vi "AOTF_NonLinKillTasks.vi"(0 "Refnum in":refnum<k21>, 1 "task out":refnum<k21>, 2 "LineOnOff[3]":bool, 3 "task out 3":refnum<k21>, 4 "LineOnOff[4]":bool, 5 "task out 7":refnum<k21>, 6 "task out 4":refnum<k21>, 7 "error in (no error)":errorcluster, 8 "LineOnOff[2]":bool, 9 "task out 6":refnum<k21>, 10 "task out 2":refnum<k21>, 11 "LineOnOff[0]":bool, 12 "LineOnOff[1]":bool, 13 "LineOnOff[5]":bool, 14 "task out 5":refnum<k21>, 15 "405Pico":refnum<k21>, 16 "LineOnOff[6]":bool, 18 "LineOnOff[7]":bool) -> (27 "error out":errorcluster)   [LabVIEW 2011]
uses:
  Variables/405Pico.vi
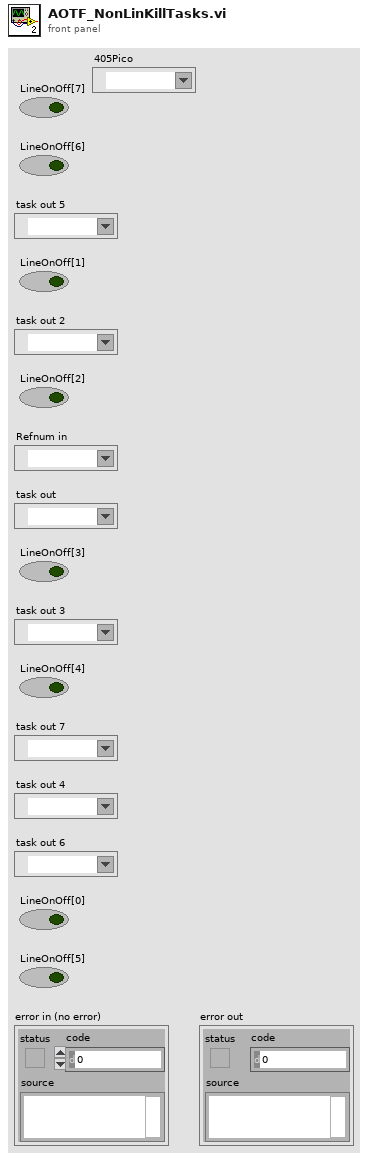
[diagram p1: front panel]
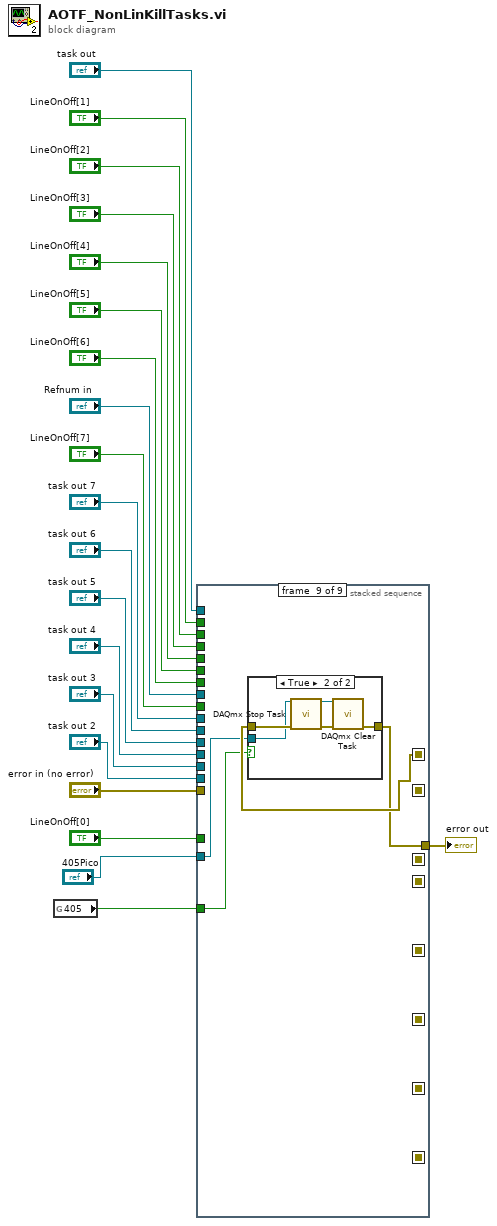
[diagram p0: block diagram]
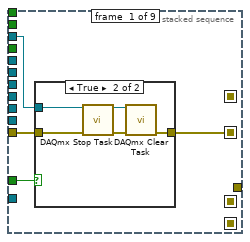
[diagram p2: hidden frame]
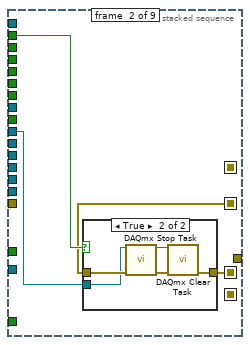
[diagram p4: hidden frame]
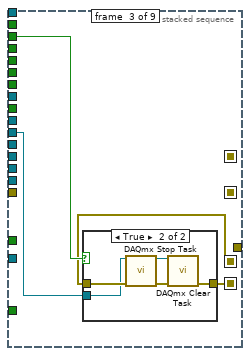
[diagram p6: hidden frame]
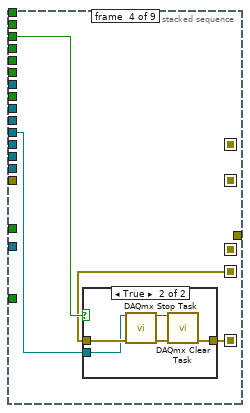
[diagram p8: hidden frame]
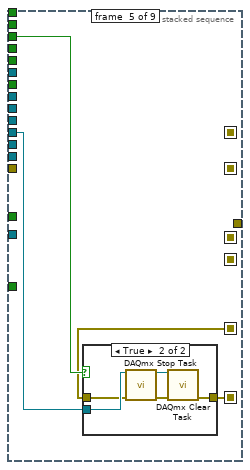
[diagram p10: hidden frame]
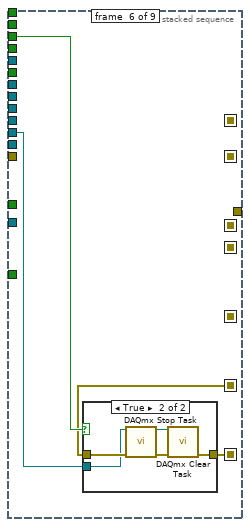
[diagram p12: hidden frame]
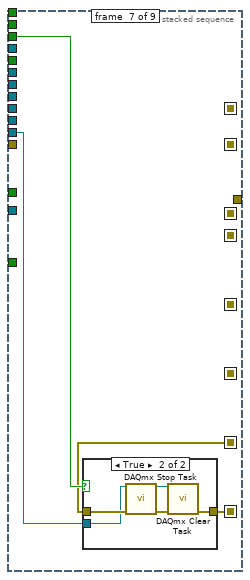
[diagram p14: hidden frame]
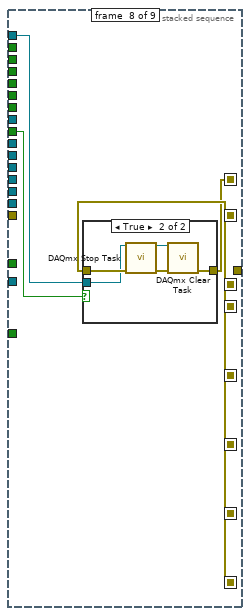
[diagram p16: hidden frame]
diagram:
  n1 = global read "405Pico.vi" "405"() -> (w2:bool)
  n2 = stacked-sequence {
    seq-local: [w21 _ _ _ _ _ _ _ _] -> [_ w32 _ _ _ _ _ _ _]
    seq-local: [_ w31 _ _ _ _ _ _ _] -> [_ _ w42 _ _ _ _ _ _]
    seq-local: [_ _ w41 _ _ _ _ _ _] -> [_ _ _ w52 _ _ _ _ _]
    seq-local: [_ _ _ w51 _ _ _ _ _] -> [_ _ _ _ w62 _ _ _ _]
    seq-local: [_ _ _ _ w61 _ _ _ _] -> [_ _ _ _ _ w72 _ _ _]
    seq-local: [_ _ _ _ _ w71 _ _ _] -> [_ _ _ _ _ _ w82 _ _]
    seq-local: [_ _ _ _ _ _ w81 _ _] -> [_ _ _ _ _ _ _ w92 _]
    seq-local: [_ _ _ _ _ _ _ w91 _] -> [_ _ _ _ _ _ _ _ w104]
    tunnel: [_ _ _ _ _ _ _ _ w103] -> w4
    tunnel: "error in (no error)" -> [w24 _ _ _ _ _ _ _ _]
    tunnel: "LineOnOff[0]" -> [w23 _ _ _ _ _ _ _ _]
    tunnel: "LineOnOff[1]" -> [_ w34 _ _ _ _ _ _ _]
    tunnel: "LineOnOff[2]" -> [_ _ w44 _ _ _ _ _ _]
    tunnel: "LineOnOff[3]" -> [_ _ _ w54 _ _ _ _ _]
    tunnel: "LineOnOff[4]" -> [_ _ _ _ w64 _ _ _ _]
    tunnel: "LineOnOff[5]" -> [_ _ _ _ _ w74 _ _ _]
    tunnel: "LineOnOff[6]" -> [_ _ _ _ _ _ w84 _ _]
    tunnel: "LineOnOff[7]" -> [_ _ _ _ _ _ _ w94 _]
    tunnel: "Refnum in" -> [w22 _ _ _ _ _ _ _ _]
    tunnel: "task out 7" -> [_ w33 _ _ _ _ _ _ _]
    tunnel: "task out 6" -> [_ _ w43 _ _ _ _ _ _]
    tunnel: "task out 5" -> [_ _ _ w53 _ _ _ _ _]
    tunnel: "task out 4" -> [_ _ _ _ w63 _ _ _ _]
    tunnel: "task out 3" -> [_ _ _ _ _ w73 _ _ _]
    tunnel: "task out 2" -> [_ _ _ _ _ _ w83 _ _]
    tunnel: "task out" -> [_ _ _ _ _ _ _ w93 _]
    tunnel: w2 -> [_ _ _ _ _ _ _ _ w102]
    tunnel: "405Pico" -> [_ _ _ _ _ _ _ _ w101]
    frame #0 {
      n3 = case shown="True" w23 {
        tunnel: [w25 w28] -> w21
        tunnel: w24 -> [w25 w27]
        tunnel: w22 -> [_ w26]
        frame False {
        }
        frame True {
          n4 = call <vilib>:"DAQmx Stop Task.vi"("task/channels in"=w26, "error in"=w27) -> ("task out"=w29:refnum<k21>, "error out"=w30:errorcluster)  [unwired: 12 in]
          n5 = call <vilib>:"DAQmx Clear Task.vi"("task in"=w29, "error in"=w30) -> ("error out"=w28:errorcluster)  [unwired: 13 in]
        }
      }
    }
    frame #1 {
      n6 = case shown="True" w34 {
        tunnel: [w35 w38] -> w31
        tunnel: w32 -> [w35 w37]
        tunnel: w33 -> [_ w36]
        frame False {
        }
        frame True {
          n7 = call <vilib>:"DAQmx Stop Task.vi"("task/channels in"=w36, "error in"=w37) -> ("task out"=w39:refnum<k21>, "error out"=w40:errorcluster)  [unwired: 12 in]
          n8 = call <vilib>:"DAQmx Clear Task.vi"("task in"=w39, "error in"=w40) -> ("error out"=w38:errorcluster)  [unwired: 13 in]
        }
      }
    }
    frame #2 {
      n9 = case shown="True" w44 {
        tunnel: [w45 w48] -> w41
        tunnel: w42 -> [w45 w47]
        tunnel: w43 -> [_ w46]
        frame False {
        }
        frame True {
          n10 = call <vilib>:"DAQmx Stop Task.vi"("task/channels in"=w46, "error in"=w47) -> ("task out"=w49:refnum<k21>, "error out"=w50:errorcluster)  [unwired: 12 in]
          n11 = call <vilib>:"DAQmx Clear Task.vi"("task in"=w49, "error in"=w50) -> ("error out"=w48:errorcluster)  [unwired: 13 in]
        }
      }
    }
    frame #3 {
      n12 = case shown="True" w54 {
        tunnel: [w55 w58] -> w51
        tunnel: w52 -> [w55 w57]
        tunnel: w53 -> [_ w56]
        frame False {
        }
        frame True {
          n13 = call <vilib>:"DAQmx Stop Task.vi"("task/channels in"=w56, "error in"=w57) -> ("task out"=w59:refnum<k21>, "error out"=w60:errorcluster)  [unwired: 12 in]
          n14 = call <vilib>:"DAQmx Clear Task.vi"("task in"=w59, "error in"=w60) -> ("error out"=w58:errorcluster)  [unwired: 13 in]
        }
      }
    }
    frame #4 {
      n15 = case shown="True" w64 {
        tunnel: [w65 w68] -> w61
        tunnel: w62 -> [w65 w66]
        tunnel: w63 -> [_ w67]
        frame False {
        }
        frame True {
          n16 = call <vilib>:"DAQmx Stop Task.vi"("task/channels in"=w67, "error in"=w66) -> ("task out"=w69:refnum<k21>, "error out"=w70:errorcluster)  [unwired: 12 in]
          n17 = call <vilib>:"DAQmx Clear Task.vi"("task in"=w69, "error in"=w70) -> ("error out"=w68:errorcluster)  [unwired: 13 in]
        }
      }
    }
    frame #5 {
      n18 = case shown="True" w74 {
        tunnel: [w75 w78] -> w71
        tunnel: w72 -> [w75 w77]
        tunnel: w73 -> [_ w76]
        frame False {
        }
        frame True {
          n19 = call <vilib>:"DAQmx Stop Task.vi"("task/channels in"=w76, "error in"=w77) -> ("task out"=w79:refnum<k21>, "error out"=w80:errorcluster)  [unwired: 12 in]
          n20 = call <vilib>:"DAQmx Clear Task.vi"("task in"=w79, "error in"=w80) -> ("error out"=w78:errorcluster)  [unwired: 13 in]
        }
      }
    }
    frame #6 {
      n21 = case shown="True" w84 {
        tunnel: [w85 w88] -> w81
        tunnel: w82 -> [w85 w87]
        tunnel: w83 -> [_ w86]
        frame False {
        }
        frame True {
          n22 = call <vilib>:"DAQmx Stop Task.vi"("task/channels in"=w86, "error in"=w87) -> ("task out"=w89:refnum<k21>, "error out"=w90:errorcluster)  [unwired: 12 in]
          n23 = call <vilib>:"DAQmx Clear Task.vi"("task in"=w89, "error in"=w90) -> ("error out"=w88:errorcluster)  [unwired: 13 in]
        }
      }
    }
    frame #7 {
      n24 = case shown="True" w94 {
        tunnel: [w95 w98] -> w91
        tunnel: w92 -> [w95 w97]
        tunnel: w93 -> [_ w96]
        frame False {
        }
        frame True {
          n25 = call <vilib>:"DAQmx Stop Task.vi"("task/channels in"=w96, "error in"=w97) -> ("task out"=w99:refnum<k21>, "error out"=w100:errorcluster)  [unwired: 12 in]
          n26 = call <vilib>:"DAQmx Clear Task.vi"("task in"=w99, "error in"=w100) -> ("error out"=w98:errorcluster)  [unwired: 13 in]
        }
      }
    }
    frame #8 {
      n27 = case shown="True" w102 {
        tunnel: [w105 w108] -> w103
        tunnel: w104 -> [w105 w107]
        tunnel: w101 -> [_ w106]
        frame False {
        }
        frame True {
          n28 = call <vilib>:"DAQmx Stop Task.vi"("task/channels in"=w106, "error in"=w107) -> ("task out"=w109:refnum<k21>, "error out"=w110:errorcluster)  [unwired: 12 in]
          n29 = call <vilib>:"DAQmx Clear Task.vi"("task in"=w109, "error in"=w110) -> ("error out"=w108:errorcluster)  [unwired: 13 in]
        }
      }
    }
  }
  "error out" <- w4
